vi "libssh2_session_set_read_timeout.vi"(8 "error in (no error)":errorcluster, 10 "read timeout in seconds (0 = default)":i32, 11 "session":T1) -> (0 "error out":errorcluster)   [LabVIEW 2013, in "libssh2.lvlib"]
doc: "Set the timeout for socket read functions on a session. Set to zero to use the default value (60 s)."
uses:
  libssh2.lvlib
  Session Refnum.ctl
  Not A Session.vi
  <vilib>/Utility/error.llb/Error Cluster From Error Code.vi
  Global Settings.vi
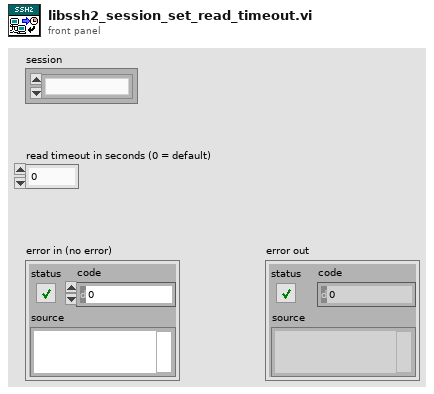
[diagram p1: front panel]
types:
  T1 = typedef "libssh2.lvlib/Session Refnum.ctl" = refnum<k1>
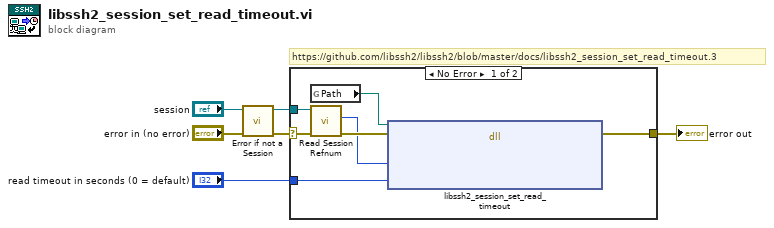
[diagram p0: block diagram]
diagram:
  # "https://github.com/libssh2/libssh2/blob/master/docs/libssh2_session_set_read_timeout.3"
  n1 = call "Error if not a Session.vi"("error in (no error)"="error in (no error)", "session"="session") -> ("error out"=w4:errorcluster, "session out"=w2:T1)  [unwired: 8 in]
  n2 = case shown="No Error" w4 {
    selector: w4 -> [w12 w14]
    tunnel: [w13 w14] -> w6
    tunnel: w2 -> [w11 _]
    tunnel: "read timeout in seconds (0 = default)" -> [w7 _]
    frame No Error {
      n3 = global read "Global Settings.vi" "Path"() -> (w8:path)
      n4 = call "Read Session Refnum.vi"("error in (no error)"=w12, "session"=w11) -> ("error out"=w10:errorcluster, "LIBSSH2_SESSION*"=w9:u64)  [unwired: 5 in, 3 out]
      n5 = dll-call lib="?" fn="libssh2_session_set_read_timeout"(path in=w8, error in=w10, "session"=w9, "timeout"=w7) -> (error out=w13:errorcluster)  [unwired: 4 in, 1 out]
    }
    frame Error {
    }
  }
  "error out" <- w6
